vi "LFO Electrical Tests.vi"() -> ()   [LabVIEW 2018]
doc: "Use this template to build a producer/consumer design pattern with events to produce queue items. Use this design pattern instead of the User Interface Event Handler pattern for user interfaces when you want to execute code asynchronously in response to an event without slowing the user interface responsiveness."
uses:
  Custom Controls/LFO State Variable.ctl
  Custom Controls/BW NF State.ctl
  Custom Controls/Vitrek State Top.ctl
  Instrumentation/Door Status Global Variable.vi
  <vilib>/DAQmx/create/channels.llb/DAQmx Create Channel (DI-Digital Input).vi
panel:
  in  "base path":path=path "F:/Departments/Mfg Production/Shares/Plant2/LFO/125332 Electrical Test"
  out "Vitrek Stop?":bool
  out "BW2 Result Indicators":T1
  out "BW1 Result Indicators":T1
  out "BW 2 Results":T2
  out "BW 1 Results":T2
  out "Raw Data ACW BW1":T3
  out "Raw Data ACW BW2":T4
  in  "Vitrek State":T5
  out "No Fire Stop?":bool
  out "BW Stop?":bool
  out "Bridgewire 2 No-Fire":waveform(dbl)(graph)
  out "Bridgewire 1 No-Fire":waveform(dbl)(graph)
  out "No-Fire Results BW1":T6
  out "No-Fire Results BW2":T6
  in  "lower resistance limit":dbl=0.13
  in  "upper resistance limit":dbl=0.25
  out "BW 2 Resistance":string
  out "BW 1 Resistance":string
  out "Model # Out":string
  out "Serial # Out":string
  in  "BW State":T7
  out "Results Table":string[][](array[string])
  out "No-Fire Result":bool
  out "configuration file path":path=path "U:/Software Development/builds/LFO Electrical Tests/LFO Electrical Test/LFO Specifications.ini"
  in  "Tab Control":enum32{"Electrical Tests"}(tab)
  in  "Reset":bool
  out "Test Status":string
  out "Results":string[][](table)
  out "BW 1 Dielectric Strength Result":u16(ring)
  out "BW 2 Dielectric Strength Result":u16(ring)
  out "BW 1 Insulation Resistance Result":u16(ring)
  out "BW 2 Insulation Resistance Result":u16(ring)
  out "BW 1 Resistance Result":u16(ring)
  out "BW 2 Resistance Result":u16(ring)
  out "BW 1 No-Fire Result":u16(ring)
  out "BW 2 No-Fire Result":u16(ring)
  in  "stop":bool
  in  "Start Vitrek":bool=TRUE
  in  "Start BW":bool=TRUE
  out "Door Status":bool
  out "Raw Data Path":path
  in  "LFO State":T8=enum."Bridgewire"
  # "LFO Electrical Tests v2.0.2"
  # "Last Updated: 8/2/2022"
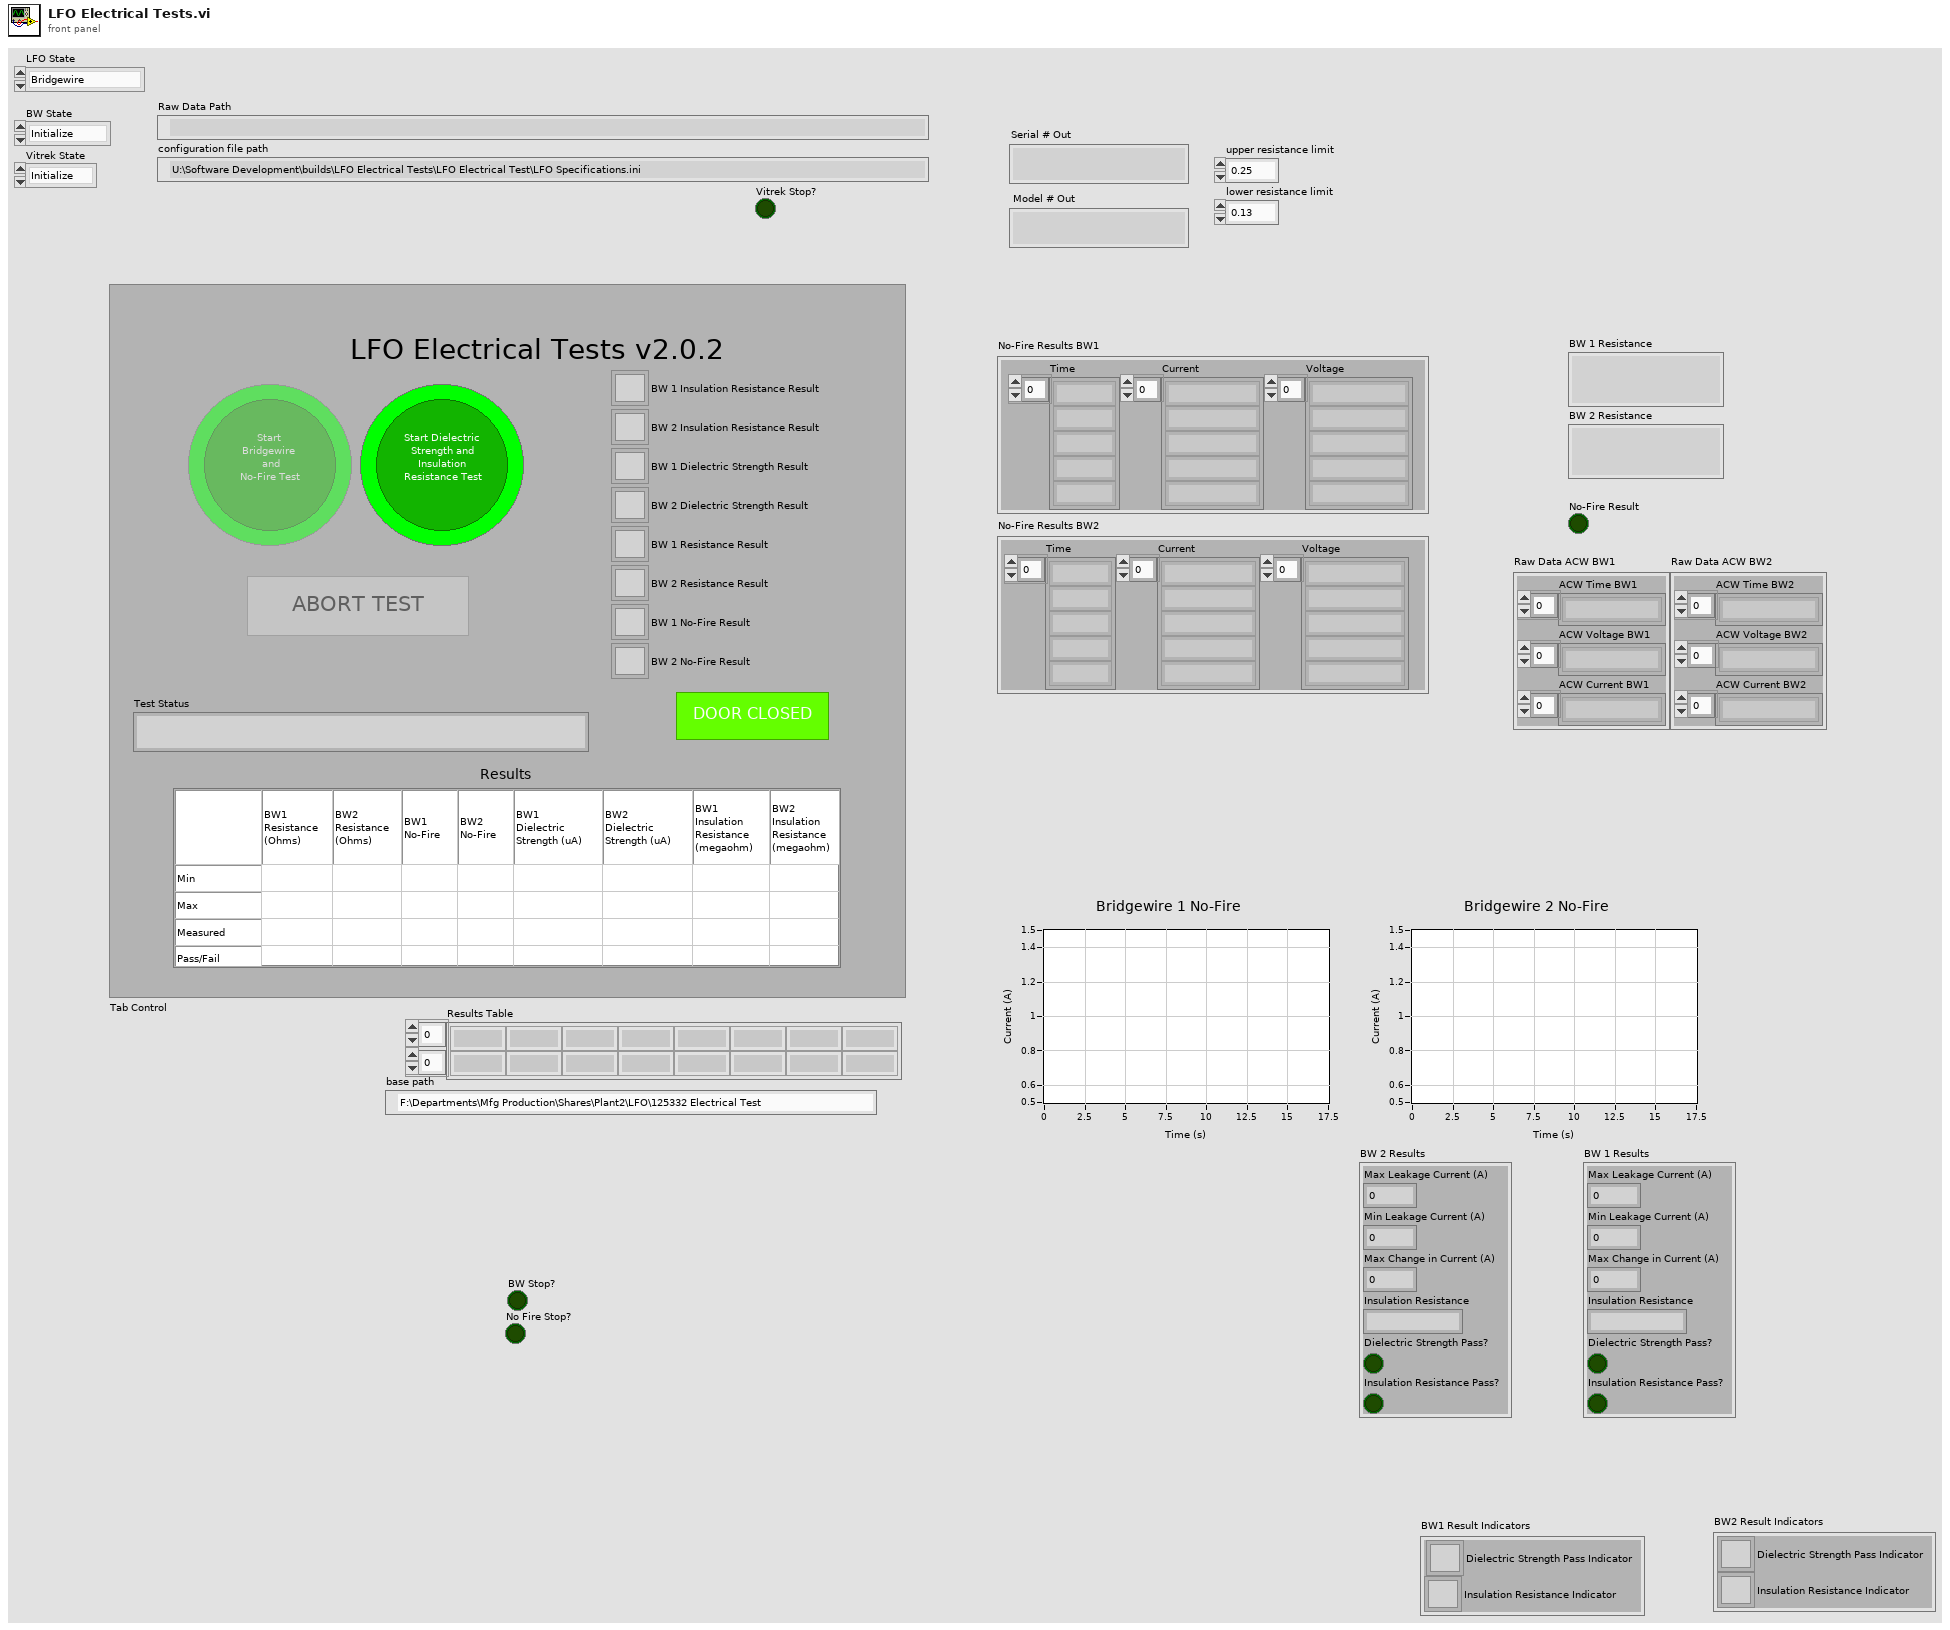
[diagram p1: front panel]
types:
  T1 = cluster{"Dielectric Strength Pass Indicator":u16, "Insulation Resistance Indicator":u16}
  T2 = cluster{"Max Leakage Current (A)":dbl, "Min Leakage Current (A)":dbl, "Max Change in Current (A)":dbl, "Dielectric Strength Pass?":bool, "Insulation Resistance Pass?":bool, "Insulation Resistance":string}
  T3 = cluster{"ACW Time BW1":string[], "ACW Voltage BW1":string[], "ACW Current BW1":string[]}
  T4 = cluster{"ACW Time BW2":string[], "ACW Voltage BW2":string[], "ACW Current BW2":string[]}
  T5 = typedef "Vitrek State Top.ctl" = enum16{"Initialize", "Run Vitrek", "End Vitrek"}
  T6 = cluster{"Current":string[], "Voltage":string[], "Time":string[]}
  T7 = typedef "BW NF State.ctl" = enum16{"Initialize", "Bridgewire Resistance", "No Fire Test", "End BW State"}
  T8 = typedef "LFO State Variable.ctl" = enum16{"Reset", "Bridgewire", "Switch Cable", "ACW and IR Test", "Report", "Exit"}
  T9 = cluster{"Instrument":string, "VISA resource name":refnum<visa-resource-name>}[]
  T10 = cluster{"BW1 Resistance (Ohms)":string, "BW2 Resistance (Ohms)":string, "BW1 No-Fire":string, "BW2 No-Fire":string, "BW1 Dielectric Strength (uA)":string, "BW2 Dielectric Strength (uA)":string, "BW1 Insulation Resistance (MOhms)":string, "BW2 Insulation Resistance (MOhms)":string}
  T11 = enum8{"Enabled", "Disabled", "Disabled and Grayed Out"}
  T12 = cluster{"BW 1 Resistance":string, "BW 2 Resistance":string, "No-Fire Results BW1":cluster{"Current":string[], "Voltage":string[], "Time":string[]}, "No-Fire Results BW2":cluster{"Current":string[], "Voltage":string[], "Time":string[]}, "ACW Results BW1":cluster{"ACW Time BW1":string[], "ACW Voltage BW1":string[], "ACW Current BW1":string[]}, "IR Results BW1":cluster{"Max Leakage Current (A)":dbl, "Min Leakage Current (A)":dbl, "Max Change in Current (A)":dbl, "Dielectric Strength Pass?":bool, "Insulation Resistance Pass?":bool, "Insulation Resistance":string}, "ACW Results BW2":cluster{"ACW Time BW2":string[], "ACW Voltage BW2":string[], "ACW Current BW2":string[]}, "IR Results BW 2":cluster{"Max Leakage Current (A)":dbl, "Min Leakage Current (A)":dbl, "Max Change in Current (A)":dbl, "Dielectric Strength Pass?":bool, "Insulation Resistance Pass?":bool, "Insulation Resistance":string}}
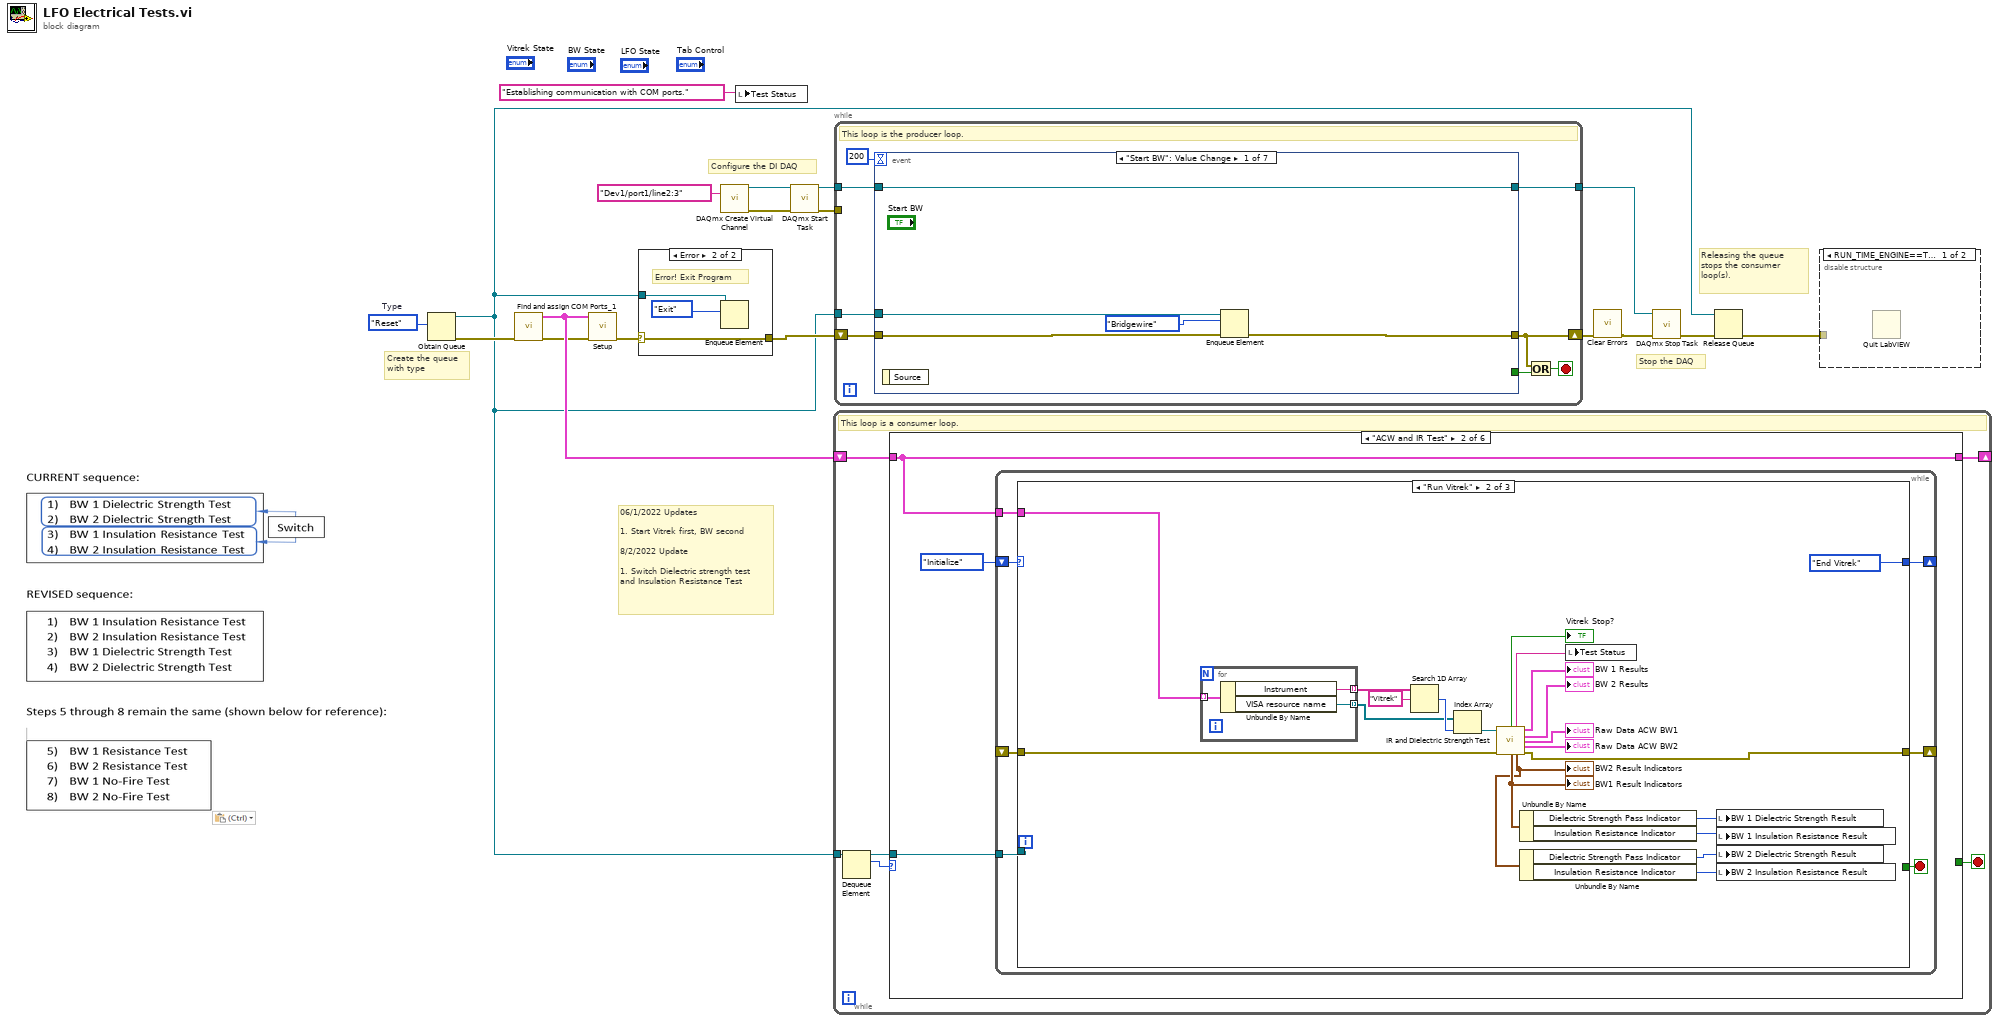
[diagram p0: block diagram]
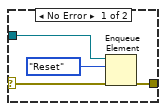
[diagram p3: hidden frame]
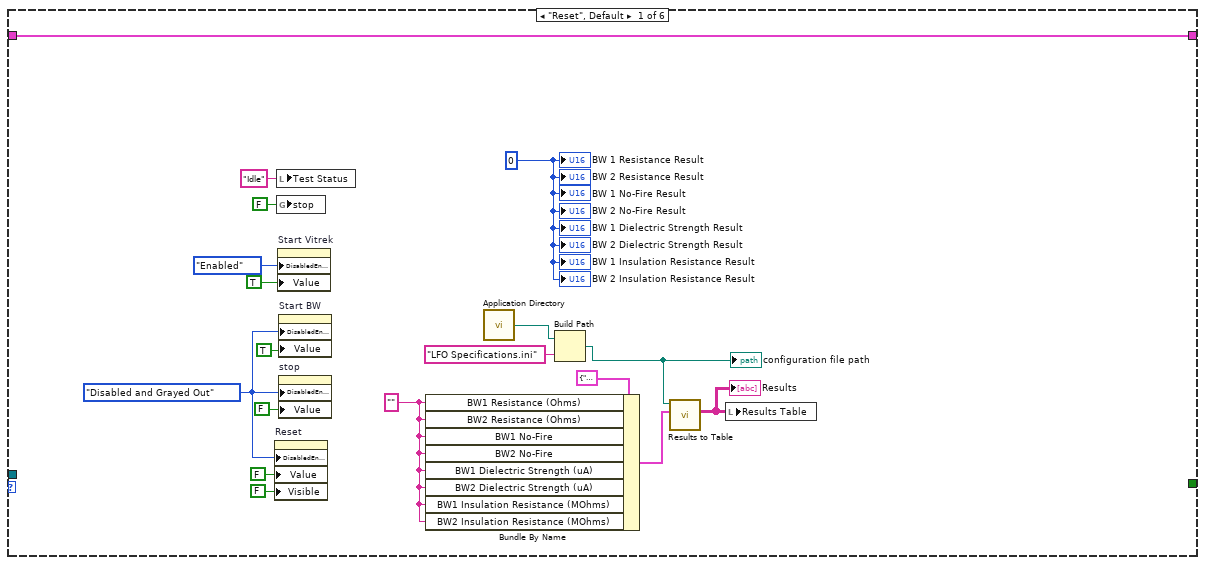
[diagram p4: hidden frame]
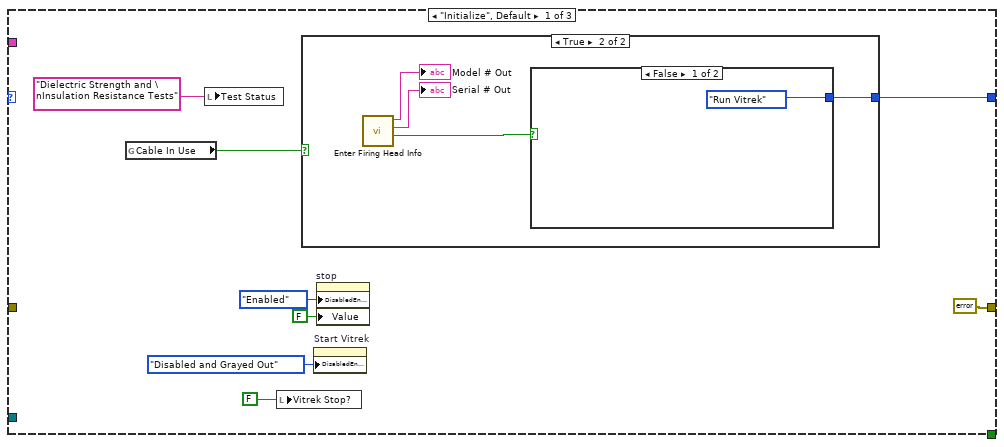
[diagram p5: hidden frame]
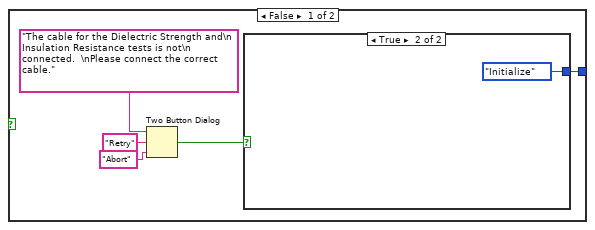
[diagram p6: hidden frame]
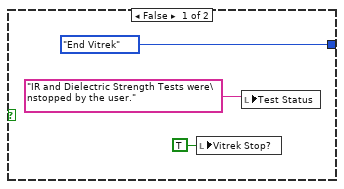
[diagram p7: hidden frame]
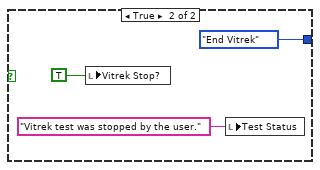
[diagram p8: hidden frame]
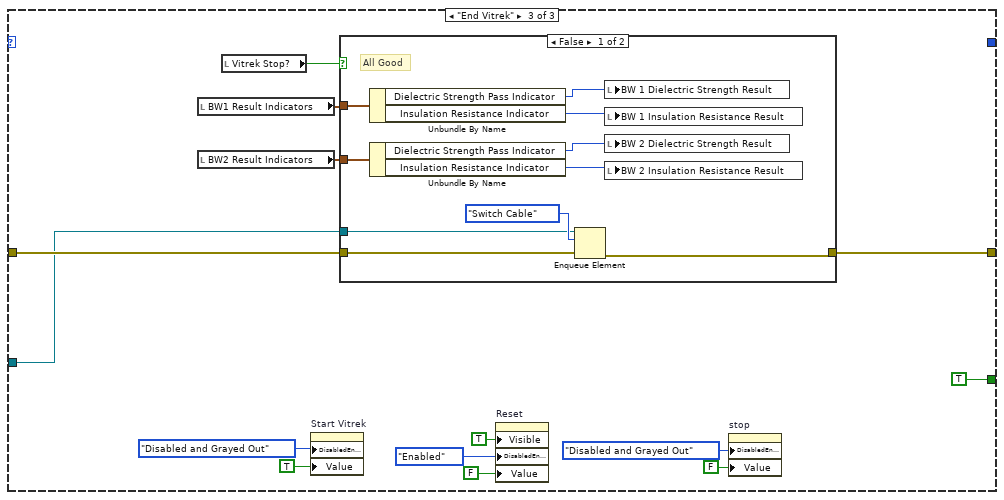
[diagram p9: hidden frame]
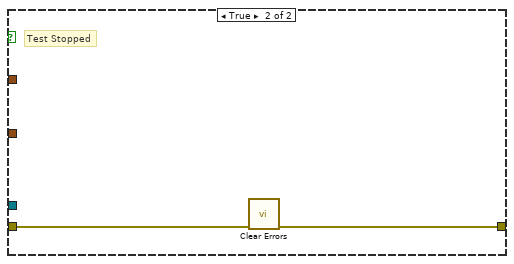
[diagram p10: hidden frame]
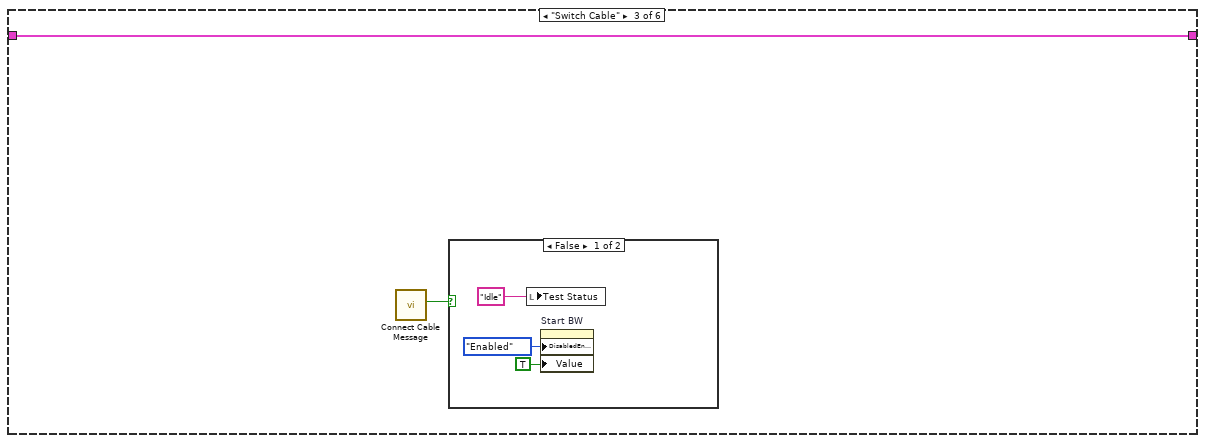
[diagram p11: hidden frame]
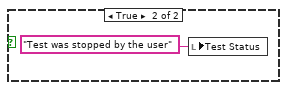
[diagram p12: hidden frame]
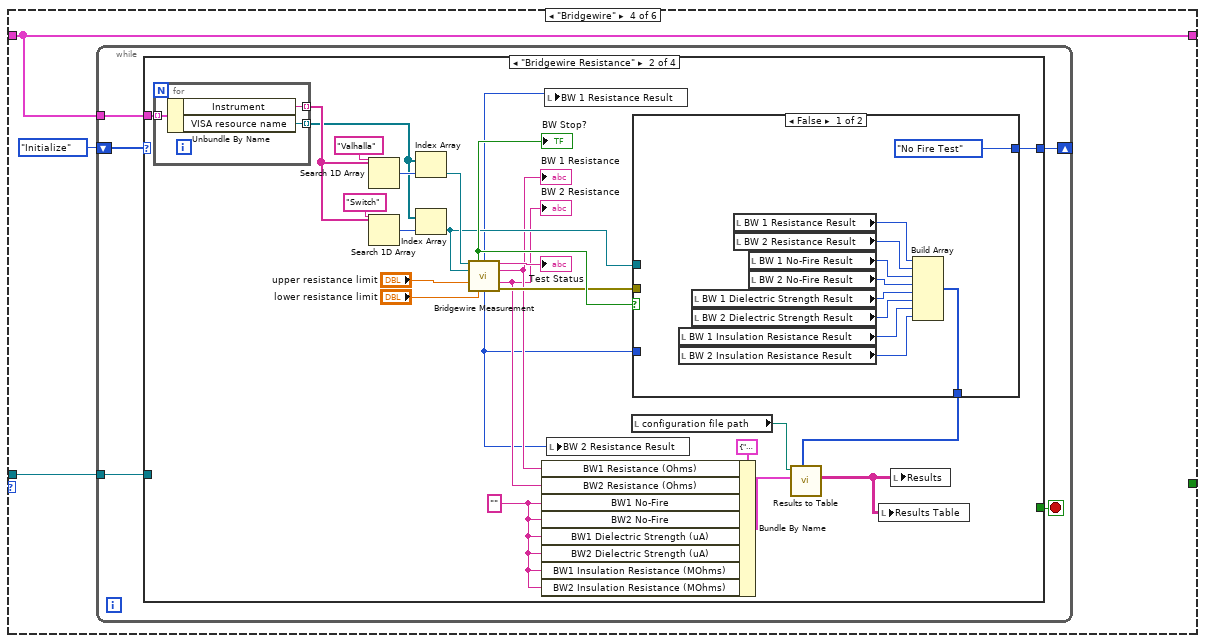
[diagram p13: hidden frame]
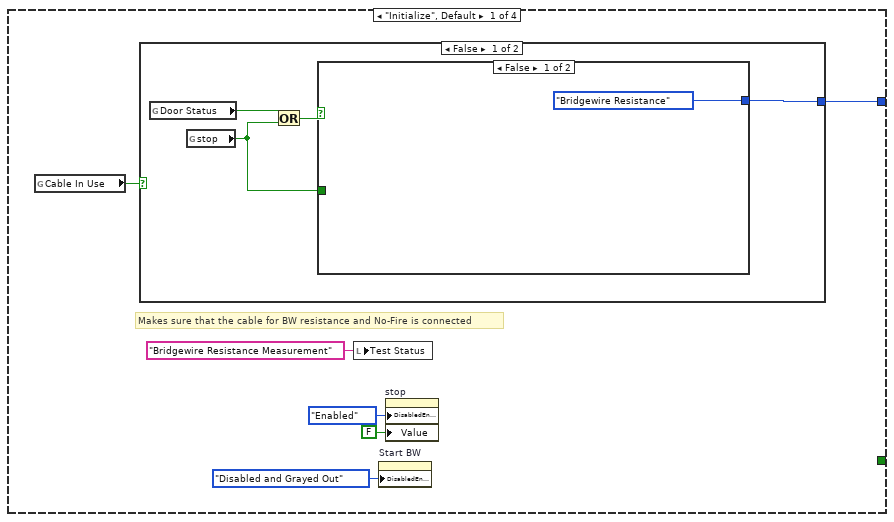
[diagram p14: hidden frame]
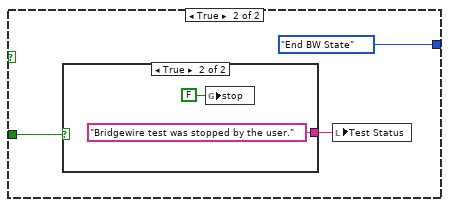
[diagram p15: hidden frame]
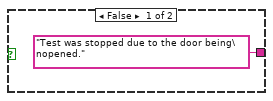
[diagram p16: hidden frame]
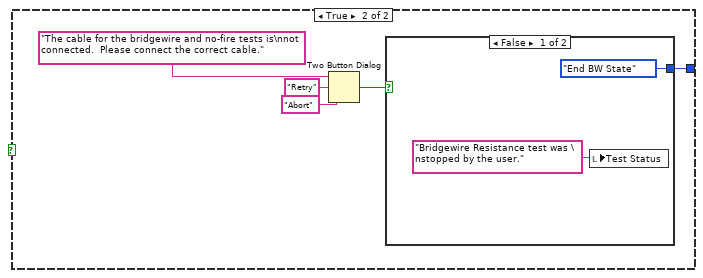
[diagram p17: hidden frame]
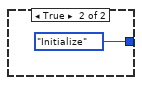
[diagram p18: hidden frame]
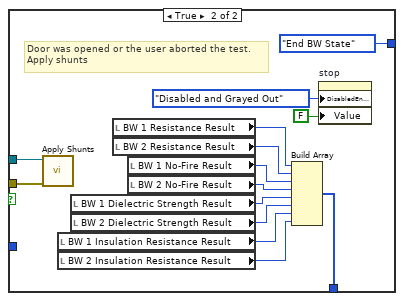
[diagram p19: hidden frame]
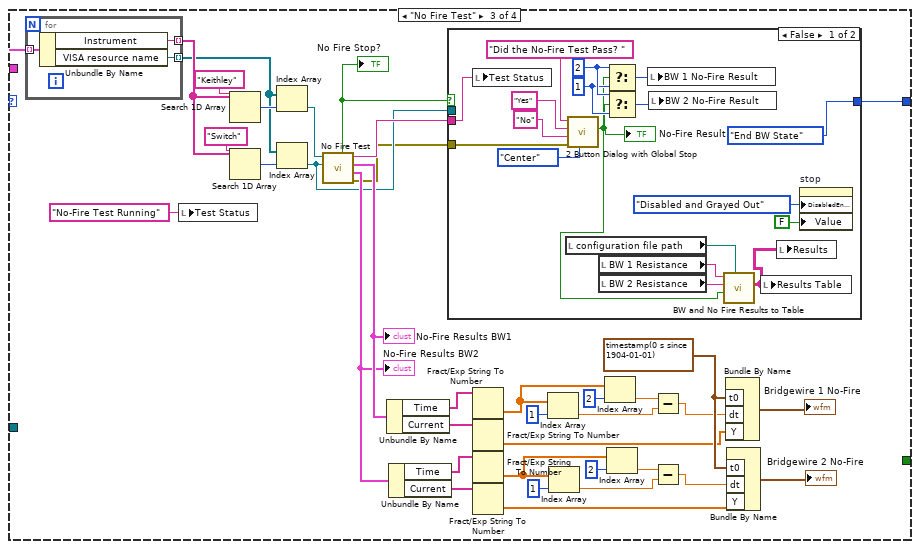
[diagram p20: hidden frame]
diagram:
  w18 = LFO_State_Variable."Reset"  # Type
  # "Stop the DAQ"
  # "Configure the DI DAQ"
  # "Create the queue\nwith type"
  # "06/1/2022 Updates\n\n1. Start Vitrek first, BW second\n\n8/2/2022 Update\n\n1. Switch Dielectric strength test\nand Insulation Resistance Test"
  # "Releasing the queue stops the consumer loop(s)."
  n1 = Obtain Queue(element data type=w18) -> (queue out=w10:refnum<queue>, error out=w11:errorcluster)  [unwired: 4 in, 1 out]
  n2 = call "Find and assign COM Ports_1.vi"("error in (no error)"=w11) -> ("error out"=w1:errorcluster, "Assigned VISA Ports"=w16:T9)  [unwired: 8 in, 1 out]
  n3 = call "Setup.vi"("error in (no error)"=w1, "Assigned VISA Ports"=w16) -> ("error out"=w6:errorcluster)  [unwired: 9 in]
  n4 = case shown="Error" w6 {
    selector: w6 -> [w21 w22]
    tunnel: [w21 w22] -> w17
    tunnel: w10 -> [w19 w24]
    frame No Error {
      n5 = Enqueue Element(queue=w19, element=LFO_State_Variable."Reset") -> ()  [unwired: 2 in, 3 out]
    }
    frame Error {
      # "Error! Exit Program"
      n6 = Enqueue Element(queue=w24, element=LFO_State_Variable."Exit") -> ()  [unwired: 2 in, 3 out]
    }
  }
  n7 = call-poly <vilib>:"DAQmx Create Virtual Channel.vi"("lines"=tag "Dev1/port1/line2:3" ("Door Status Input")) -> ("task out"=w8:refnum<k21>, "error out"=w9:errorcluster)  [unwired: 13 in]
  n8 = local write "Test Status"("Establishing communication with COM ports." ("Test Status")) -> ()
  n9 = call <vilib>:"DAQmx Start Task.vi"("task/channels in"=w8, "error in"=w9) -> ("task out"=w15:refnum<k21>, "error out"=w2:errorcluster)  [unwired: 12 in]
  n10 = while {
    tunnel: w10 -> [w30]
    shift-right: [w26] -> _
    shift-left: w16 -> [w27]
    stop <- w28 stop-if-true
    # "This loop is a consumer loop."
    n11 = Dequeue Element(queue=w30) -> (queue out=w25:refnum<queue>, element=w29:T8)  [unwired: 2 in, 2 out]
    n12 = case shown="\"ACW and IR Test\"" w29 {
      tunnel: w27 -> [w48 w50 w135 w142 w353 w354]
      tunnel: [_ _ _ _ _ TRUE] -> w28
      tunnel: [w48 w50 w135 w142 w353 w354] -> w26
      tunnel: w25 -> [_ w49 _ w140 _ _]
      frame "Reset", Default {
        w32 = u16 0 ("BW 1 Resistance Result")
        w31 = T11."Disabled and Grayed Out" ("Disabled")
        w41 = "" ("BW1 Resistance (Ohms)")
        n13 = property on="Reset" class="Bool (strict)"("DisabledEnum"=w31, "Value"=FALSE ("stop"), "Visible"=FALSE) -> ()  [unwired: 2 in, 2 out]
        n14 = local write "Test Status"("Idle" ("Test Status")) -> ()
        n15 = global write "Door Status Global Variable.vi" "stop"(FALSE ("stop")) -> ()
        n16 = property on="Start Vitrek" class="Bool (strict)"("DisabledEnum"=T11."Enabled" ("Disabled"), "Value"=TRUE ("stop")) -> ()  [unwired: 2 in, 2 out]
        n17 = property on="Start BW" class="Bool (strict)"("DisabledEnum"=w31, "Value"=TRUE ("stop")) -> ()  [unwired: 2 in, 2 out]
        n18 = property on="stop" class="Bool (strict)"("DisabledEnum"=w31, "Value"=FALSE ("stop")) -> ()  [unwired: 2 in, 2 out]
        n19 = Bundle By Name(cluster=T10 {"BW1 Resistance (Ohms)"="4870 ", "BW2 Resistance (Ohms)"="4870 ", "BW1 No-Fire"="4870 ", "BW2 No-Fire"="4870 ", "BW1 Dielectric Strength (uA)"="4870 ", "BW2 Dielectric Strength (uA)"="4870 ", "BW1 Insulation Resistance (MOhms)"="4870 ", "BW2 Insulation Resistance (MOhms)"="4870 "} ("Test Results"), "BW1 Resistance (Ohms)"=w41, "BW2 Resistance (Ohms)"=w41, "BW1 No-Fire"=w41, "BW2 No-Fire"=w41, "BW1 Dielectric Strength (uA)"=w41, "BW2 Dielectric Strength (uA)"=w41, "BW1 Insulation Resistance (MOhms)"=w41, "BW2 Insulation Resistance (MOhms)"=w41) -> (w43:T10)
        n20 = call <vilib>:"Application Directory.vi"() -> ("Application Directory"=w38:path)
        n21 = Build Path(base path=w38, name or relative path="LFO Specifications.ini") -> (appended path=w36:path)
        "configuration file path" <- w36
        n22 = call "Results to Table.vi"("Test Results"=w43, "configuration file path"=w36) -> ("Results Table"=w39:string[][])  [unwired: 8 in, 1 out]
        "Results" <- w39
        n23 = local write "Results Table"(w39) -> ()
        "BW 1 Dielectric Strength Result" <- w32
        "BW 2 Dielectric Strength Result" <- w32
        "BW 1 Insulation Resistance Result" <- w32
        "BW 2 Insulation Resistance Result" <- w32
        "BW 1 Resistance Result" <- w32
        "BW 2 Resistance Result" <- w32
        "BW 1 No-Fire Result" <- w32
        "BW 2 No-Fire Result" <- w32
      }
      frame "ACW and IR Test" {
        n24 = while {
          shift-right: [w57] -> _
          shift-left: Vitrek_State_Top."Initialize" ("Vitrek State") -> [w58]
          tunnel: w50 -> [w56]
          shift-right: [w55] -> _
          shift-left: _ -> [w54]
          tunnel: w49 -> [w52]
          stop <- w53 stop-if-true
          n25 = case shown="\"Run Vitrek\"" w58 {
            tunnel: [w66 Vitrek_State_Top."End Vitrek" ("Vitrek State") _] -> w57
            tunnel: w56 -> [_ w100 _]
            tunnel: [errorcluster {"status"=FALSE, "code"=0, "source"=""} ("error in (no error)") w92 w108] -> w55
            tunnel: w54 -> [_ w98 w121]
            tunnel: [_ _ TRUE] -> w53
            tunnel: w52 -> [_ _ w109]
            frame "Initialize", Default {
              n26 = global read "Door Status Global Variable.vi" "Cable In Use"() -> (w60:bool)
              n27 = local write "Test Status"("Dielectric Strength and \nInsulation Resistance Tests" ("Test Status")) -> ()
              n28 = local write "Vitrek Stop?"(FALSE ("Vitrek Init Stop?")) -> ()
              n29 = case shown="True" w60 {
                tunnel: [w68 w79] -> w66
                frame False {
                  n30 = Two Button Dialog(message="The cable for the Dielectric Strength and\n Insulation Resistance tests is not\n connected.  \nPlease connect the correct cable.", 1:"Abort" ("F button name (\"Cancel\")"), 2:"Retry" ("T button name (\"OK\")")) -> (T button?=w67:bool)
                  n31 = case shown="True" w67 {
                    tunnel: [Vitrek_State_Top."End Vitrek" ("Vitrek State") Vitrek_State_Top."Initialize" ("Vitrek State")] -> w68
                    frame False {
                      n32 = local write "Vitrek Stop?"(TRUE ("Vitrek Stop?")) -> ()
                      n33 = local write "Test Status"("IR and Dielectric Strength Tests were\nstopped by the user." ("Test Status")) -> ()
                    }
                    frame True {
                    }
                  }
                }
                frame True {
                  n34 = call "Enter Firing Head Info.vi"() -> ("Abort Test?"=w76:bool, "Serial # Out"=→"Serial # Out":string, "Model # Out"=→"Model # Out":string)  [unwired: 7 in, 1 out]
                  n35 = case shown="False" w76 {
                    tunnel: [Vitrek_State_Top."Run Vitrek" ("Vitrek State") Vitrek_State_Top."End Vitrek" ("Vitrek State")] -> w79
                    frame False {
                    }
                    frame True {
                      n36 = local write "Vitrek Stop?"(TRUE ("Vitrek Init Stop?")) -> ()
                      n37 = local write "Test Status"("Vitrek test was stopped by the user." ("Test Status")) -> ()
                    }
                  }
                }
              }
              n38 = property on="Start Vitrek" class="Bool (strict)"("DisabledEnum"=T11."Disabled and Grayed Out" ("Disabled")) -> ()  [unwired: 2 in, 2 out]
              n39 = property on="stop" class="Bool (strict)"("DisabledEnum"=T11."Enabled" ("Disabled"), "Value"=FALSE ("stop")) -> ()  [unwired: 2 in, 2 out]
            }
            frame "Run Vitrek" {
              n40 = for {
                tunnel: w100 -> [w107] mode=indexing
                tunnel: [w106] -> w102 mode=indexing
                tunnel: [w105] -> w101 mode=indexing
                n41 = Unbundle By Name(w107) -> ("Instrument"=w106:string, "VISA resource name"=w105:refnum<visa-resource-name>)
              }
              n42 = Search 1D Array(1D array=w102, element="Vitrek") -> (index of element=w103:i32)  [unwired: 1 in]
              n43 = Index Array(array=w101, index=w103) -> (element=w90:refnum<visa-resource-name>)
              n44 = call "IR and Dielectric Strength Test.vi"("VISA resource name in"=w90, "error in (no error)"=w98) -> (2:"Stop Status"=→"Vitrek Stop?":bool, 3:"Stop Status"=w96:string, "BW 1 Results"=→"BW 1 Results":T2, "BW 2 Results"=→"BW 2 Results":T2, "Raw Data ACW BW1"=→"Raw Data ACW BW1":T3, "Raw Data ACW BW2"=→"Raw Data ACW BW2":T4, "BW1 Result Indicators"=w85:T1, "BW2 Result Indicators"=w84:T1, "error out"=w92:errorcluster)  [unwired: 5 in]
              "BW2 Result Indicators" <- w84
              "BW1 Result Indicators" <- w85
              n45 = Unbundle By Name(w85) -> ("Dielectric Strength Pass Indicator"=w87:u16, "Insulation Resistance Indicator"=w86:u16)
              n46 = Unbundle By Name(w84) -> ("Dielectric Strength Pass Indicator"=w89:u16, "Insulation Resistance Indicator"=w88:u16)
              n47 = local write "Test Status"(w96) -> ()
              n48 = local write "BW 1 Dielectric Strength Result"(w87) -> ()
              n49 = local write "BW 1 Insulation Resistance Result"(w86) -> ()
              n50 = local write "BW 2 Dielectric Strength Result"(w89) -> ()
              n51 = local write "BW 2 Insulation Resistance Result"(w88) -> ()
            }
            frame "End Vitrek" {
              n52 = local read "BW1 Result Indicators"() -> (w111:T1)
              n53 = local read "BW2 Result Indicators"() -> (w110:T1)
              n54 = local read "Vitrek Stop?"() -> (w112:bool)
              n55 = property on="Start Vitrek" class="Bool (strict)"("DisabledEnum"=T11."Disabled and Grayed Out" ("Disabled"), "Value"=TRUE ("stop")) -> ()  [unwired: 2 in, 2 out]
              n56 = case shown="False" w112 {
                tunnel: w110 -> [w131 _]
                tunnel: w111 -> [w130 _]
                tunnel: [w122 w132] -> w108
                tunnel: w121 -> [w123 w133]
                tunnel: w109 -> [w124 _]
                frame False {
                  # "All Good"
                  n57 = Unbundle By Name(w130) -> ("Dielectric Strength Pass Indicator"=w129:u16, "Insulation Resistance Indicator"=w128:u16)
                  n58 = Unbundle By Name(w131) -> ("Dielectric Strength Pass Indicator"=w127:u16, "Insulation Resistance Indicator"=w126:u16)
                  n59 = Enqueue Element(queue=w124, element=LFO_State_Variable."Switch Cable", error in (no error)=w123) -> (error out=w122:errorcluster)  [unwired: 1 in, 2 out]
                  n60 = local write "BW 1 Dielectric Strength Result"(w129) -> ()
                  n61 = local write "BW 1 Insulation Resistance Result"(w128) -> ()
                  n62 = local write "BW 2 Dielectric Strength Result"(w127) -> ()
                  n63 = local write "BW 2 Insulation Resistance Result"(w126) -> ()
                }
                frame True {
                  # "Test Stopped"
                  n64 = call <vilib>:"Clear Errors.vi"("error in (no error)"=w133) -> ("error out"=w132:errorcluster)  [unwired: 5 in, 1 out]
                }
              }
              n65 = property on="Reset" class="Bool (strict)"("Visible"=TRUE, "DisabledEnum"=T11."Enabled" ("Disabled"), "Value"=FALSE ("Start BW")) -> ()  [unwired: 2 in, 2 out]
              n66 = property on="stop" class="Bool (strict)"("DisabledEnum"=T11."Disabled and Grayed Out" ("Disabled"), "Value"=FALSE ("Start BW")) -> ()  [unwired: 2 in, 2 out]
            }
          }
        }
      }
      frame "Switch Cable" {
        n67 = call "Connect Cable Message.vi"() -> ("Aborted?"=w134:bool)  [unwired: 10 in, 1 out]
        n68 = case shown="False" w134 {
          frame False {
            n69 = local write "Test Status"("Idle" ("Test Status")) -> ()
            n70 = property on="Start BW" class="Bool (strict)"("DisabledEnum"=T11."Enabled" ("Disabled"), "Value"=TRUE ("Start BW")) -> ()  [unwired: 2 in, 2 out]
          }
          frame True {
            n71 = local write "Test Status"("Test was stopped by the user" ("Test Status")) -> ()
          }
        }
      }
      frame "Bridgewire" {
        n72 = while {
          shift-right: [w146] -> _
          shift-left: BW_NF_State."Initialize" ("BW State") -> [w147]
          tunnel: w142 -> [w145]
          tunnel: w140 -> [w143]
          stop <- w144 stop-if-true
          n73 = case shown="\"Bridgewire Resistance\"" w147 {
            tunnel: [w153 w184 w235 _] -> w146
            tunnel: w145 -> [_ w189 w241 _]
            tunnel: [_ _ _ TRUE] -> w144
            tunnel: w143 -> [_ _ _ w294]
            frame "Initialize", Default {
              # "Makes sure that the cable for BW resistance and No-Fire is connected"
              n74 = global read "Door Status Global Variable.vi" "Cable In Use"() -> (w152:bool)
              n75 = case shown="False" w152 {
                tunnel: [w154 w166] -> w153
                frame False {
                  n76 = global read "Door Status Global Variable.vi" "Door Status"() -> (w157:bool)
                  n77 = global read "Door Status Global Variable.vi" "stop"() -> (w156:bool)
                  n78 = Or(x=w157, y=w156) -> (x .or. y?=w155:bool)
                  n79 = case shown="False" w155 {
                    tunnel: w156 -> [_ w161]
                    tunnel: [BW_NF_State."Bridgewire Resistance" ("BW State") BW_NF_State."End BW State" ("BW State")] -> w154
                    frame False {
                    }
                    frame True {
                      n80 = case shown="True" w161 {
                        tunnel: ["Test was stopped due to the door being\nopened." ("Test Status") "Bridgewire test was stopped by the user." ("Test Status")] -> w160
                        frame False {
                        }
                        frame True {
                          n81 = global write "Door Status Global Variable.vi" "stop"(FALSE ("stop")) -> ()
                        }
                      }
                      n82 = local write "Test Status"(w160) -> ()
                    }
                  }
                }
                frame True {
                  n83 = Two Button Dialog(message="The cable for the bridgewire and no-fire tests is\nnot connected.  Please connect the correct cable.", 1:"Abort" ("F button name (\"Cancel\")"), 2:"Retry" ("T button name (\"OK\")")) -> (T button?=w165:bool)
                  n84 = case shown="False" w165 {
                    tunnel: [BW_NF_State."End BW State" ("BW State") BW_NF_State."Initialize" ("BW State")] -> w166
                    frame False {
                      n85 = local write "Test Status"("Bridgewire Resistance test was \nstopped by the user." ("Test Status")) -> ()
                    }
                    frame True {
                    }
                  }
                }
              }
              n86 = local write "Test Status"("Bridgewire Resistance Measurement" ("Test Status")) -> ()
              n87 = property on="Start BW" class="Bool (strict)"("DisabledEnum"=T11."Disabled and Grayed Out" ("Disabled")) -> ()  [unwired: 2 in, 2 out]
              n88 = property on="stop" class="Bool (strict)"("DisabledEnum"=T11."Enabled" ("Disabled"), "Value"=FALSE ("stop")) -> ()  [unwired: 2 in, 2 out]
            }
            frame "Bridgewire Resistance" {
              w176 = "" ("BW1 No-Fire")
              n89 = for {
                tunnel: w189 -> [w224] mode=indexing
                tunnel: [w223] -> w190 mode=indexing
                tunnel: [w222] -> w188 mode=indexing
                n90 = Unbundle By Name(w224) -> ("Instrument"=w223:string, "VISA resource name"=w222:refnum<visa-resource-name>)
              }
              n91 = Search 1D Array(1D array=w190, element="Valhalla") -> (index of element=w193:i32)  [unwired: 1 in]
              n92 = Search 1D Array(1D array=w190, element="Switch") -> (index of element=w191:i32)  [unwired: 1 in]
              n93 = Index Array(array=w188, index=w193) -> (element=w187:refnum<visa-resource-name>)
              n94 = Index Array(array=w188, index=w191) -> (element=w183:refnum<visa-resource-name>)
              n95 = call "Bridgewire Measurement.vi"("Valhalla Resource Name"=w187, "Switch Resource Name"=w183, "upper resistance limit"="upper resistance limit", "lower resistance limit"="lower resistance limit") -> ("Stop Status"=w186:bool, "BW1 Resistance Result"=w173:u16, "Test Status"=→"Test Status":string, "BW 1 Resistance"=w179:string, "BW 2 Resistance"=w178:string, "BW2 Resistance Result"=w174:u16, "error out"=w185:errorcluster)  [unwired: 3 in, 2 out]
              "BW 1 Resistance" <- w179
              "BW 2 Resistance" <- w178
              "BW Stop?" <- w186
              n96 = Bundle By Name(cluster=T10 {"BW1 Resistance (Ohms)"="4870 ", "BW2 Resistance (Ohms)"="4870 ", "BW1 No-Fire"="4870 ", "BW2 No-Fire"="4870 ", "BW1 Dielectric Strength (uA)"="4870 ", "BW2 Dielectric Strength (uA)"="4870 ", "BW1 Insulation Resistance (MOhms)"="4870 ", "BW2 Insulation Resistance (MOhms)"="4870 "} ("Test Results"), "BW1 Resistance (Ohms)"=w179, "BW2 Resistance (Ohms)"=w178, "BW1 No-Fire"=w176, "BW2 No-Fire"=w176, "BW1 Dielectric Strength (uA)"=w176, "BW2 Dielectric Strength (uA)"=w176, "BW1 Insulation Resistance (MOhms)"=w176, "BW2 Insulation Resistance (MOhms)"=w176) -> (w181:T10)
              n97 = local write "BW 1 Resistance Result"(w173) -> ()
              n98 = local write "BW 2 Resistance Result"(w174) -> ()
              n99 = local read "configuration file path"() -> (w180:path)
              n100 = case shown="False" w186 {
                tunnel: w185 -> [_ w219]
                tunnel: [BW_NF_State."No Fire Test" ("BW State") BW_NF_State."End BW State" ("BW State")] -> w184
                tunnel: w183 -> [_ w217]
                tunnel: [w198 w208] -> w175
                tunnel: w174 -> [_ _]
                frame False {
                  n101 = local read "BW 1 Insulation Resistance Result"() -> (w200:u16)
                  n102 = local read "BW 2 Insulation Resistance Result"() -> (w199:u16)
                  n103 = local read "BW 1 Dielectric Strength Result"() -> (w202:u16)
                  n104 = local read "BW 2 Dielectric Strength Result"() -> (w201:u16)
                  n105 = local read "BW 1 Resistance Result"() -> (w206:u16)
                  n106 = local read "BW 2 Resistance Result"() -> (w205:u16)
                  n107 = local read "BW 1 No-Fire Result"() -> (w204:u16)
                  n108 = local read "BW 2 No-Fire Result"() -> (w203:u16)
                  n109 = Build Array(w206, w205, w204, w203, w202, w201, w200, w199) -> (w198:u16[])
                }
                frame True {
                  # "Door was opened or the user aborted the test.\nApply shunts"
                  n110 = call "Apply Shunts.vi"("error in (no error)"=w219, "VISA Refnum in"=w217) -> ()  [unwired: 9 in, 1 out]
                  n111 = local read "BW 1 Insulation Resistance Result"() -> (w210:u16)
                  n112 = local read "BW 2 Insulation Resistance Result"() -> (w209:u16)
                  n113 = local read "BW 1 Dielectric Strength Result"() -> (w212:u16)
                  n114 = local read "BW 2 Dielectric Strength Result"() -> (w211:u16)
                  n115 = local read "BW 1 Resistance Result"() -> (w216:u16)
                  n116 = local read "BW 2 Resistance Result"() -> (w215:u16)
                  n117 = local read "BW 1 No-Fire Result"() -> (w214:u16)
                  n118 = local read "BW 2 No-Fire Result"() -> (w213:u16)
                  n119 = Build Array(w216, w215, w214, w213, w212, w211, w210, w209) -> (w208:u16[])
                  n120 = property on="stop" class="Bool (strict)"("DisabledEnum"=T11."Disabled and Grayed Out" ("Disabled"), "Value"=FALSE ("Start BW")) -> ()  [unwired: 2 in, 2 out]
                }
              }
              n121 = call "Results to Table.vi"("Result Indicators"=w175, "Test Results"=w181, "configuration file path"=w180) -> ("Results Table"=w177:string[][])  [unwired: 7 in, 1 out]
              n122 = local write "Results Table"(w177) -> ()
              n123 = local write "Results"(w177) -> ()
            }
            frame "No Fire Test" {
              w254 = timestamp(0 s since 1904-01-01) ("t0")
              n124 = for {
                tunnel: w241 -> [w288] mode=indexing
                tunnel: [w287] -> w243 mode=indexing
                tunnel: [w286] -> w242 mode=indexing
                n125 = Unbundle By Name(w288) -> ("Instrument"=w287:string, "VISA resource name"=w286:refnum<visa-resource-name>)
              }
              n126 = local write "Test Status"("No-Fire Test Running" ("Test Status")) -> ()
              n127 = Search 1D Array(1D array=w243, element="Keithley") -> (index of element=w246:i32)  [unwired: 1 in]
              n128 = Search 1D Array(1D array=w243, element="Switch") -> (index of element=w244:i32)  [unwired: 1 in]
              n129 = Index Array(array=w242, index=w246) -> (element=w240:refnum<visa-resource-name>)
              n130 = Index Array(array=w242, index=w244) -> (element=w237:refnum<visa-resource-name>)
              n131 = call "No Fire Test.vi"("Switch Resource Name"=w237, "Keithley Resource Name"=w240) -> ("error out"=w236:errorcluster, "No-Fire Results BW2"=w248:T6, "No-Fire Results BW1"=w249:T6, "Test Status"=w238:string, "Stop Status"=w239:bool)  [unwired: 5 in]
              "No-Fire Results BW2" <- w248
              "No-Fire Results BW1" <- w249
              "No Fire Stop?" <- w239
              n132 = Unbundle By Name(w249) -> ("Time"=w260:string[], "Current"=w259:string[])
              n133 = Unbundle By Name(w248) -> ("Time"=w258:string[], "Current"=w257:string[])
              n134 = case shown="False" w239 {
                tunnel: w236 -> [w275 w284]
                tunnel: w238 -> [w270 w285]
                tunnel: w237 -> [_ w283]
                tunnel: [BW_NF_State."End BW State" ("BW State") BW_NF_State."End BW State" ("BW State")] -> w235
                frame False {
                  w277 = u16 1 ("BW 1 Resistance Result")
                  w279 = u16 2 ("BW 1 Resistance Result")
                  n135 = local write "Test Status"(w270) -> ()
                  n136 = local read "configuration file path"() -> (w264:path)
                  n137 = call "2 Button Dialog with Global Stop.vi"("Text.Justification"=enum16{"Left", "Center", "Right"}."Center", "error in (no error)"=w275, "F Button Name (\"CANCEL\")"="No" ("F button name (\"Cancel\")"), "T Button Name (\"OK\")"="Yes" ("T button name (\"OK\")"), "Dialog Message"="Did the No-Fire Test Pass? " ("message")) -> ("result"=w262:bool)  [unwired: 4 in, 2 out]
                  "No-Fire Result" <- w262
                  n138 = local read "BW 1 Resistance"() -> (w265:string)
                  n139 = local read "BW 2 Resistance"() -> (w266:string)
                  n140 = Select(t=w279, s=w262, f=w277) -> (s? t:f=w278:u16)
                  n141 = Select(t=w279, s=w262, f=w277) -> (s? t:f=w276:u16)
                  n142 = local write "BW 1 No-Fire Result"(w278) -> ()
                  n143 = local write "BW 2 No-Fire Result"(w276) -> ()
                  n144 = call "BW and No Fire Results to Table.vi"("configuration file path"=w264, "No-Fire Result"=w262, "BW 2 Resistance"=w266, "BW 1 Resistance"=w265) -> ("Results Table"=w263:string[][])  [unwired: 6 in, 1 out]
                  n145 = local write "Results Table"(w263) -> ()
                  n146 = local write "Results"(w263) -> ()
                  n147 = property on="stop" class="Bool (strict)"("DisabledEnum"=T11."Disabled and Grayed Out" ("Disabled"), "Value"=FALSE ("Start BW")) -> ()  [unwired: 2 in, 2 out]
                }
                frame True {
                  # "Door was opened or the user \naborted the test.\nApply shunts and initialize \ncontrols"
                  n148 = local write "Test Status"(w285) -> ()
                  n149 = call "Apply Shunts.vi"("error in (no error)"=w284, "VISA Refnum in"=w283) -> ()  [unwired: 9 in, 1 out]
                  n150 = property on="stop" class="Bool (strict)"("DisabledEnum"=T11."Disabled and Grayed Out" ("Disabled"), "Value"=FALSE ("Start BW")) -> ()  [unwired: 2 in, 2 out]
                }
              }
              n151 = Fract/Exp String To Number(string=w260) -> (number=w231:dbl[])  [unwired: 3 in, 1 out]
              n152 = Fract/Exp String To Number(string=w259) -> (number=w252:dbl[])  [unwired: 3 in, 1 out]
              n153 = Fract/Exp String To Number(string=w258) -> (number=w232:dbl[])  [unwired: 3 in, 1 out]
              n154 = Fract/Exp String To Number(string=w257) -> (number=w255:dbl[])  [unwired: 3 in, 1 out]
              n155 = Index Array(array=w231, index=1) -> (element=w228:dbl)
              n156 = Index Array(array=w232, index=1) -> (element=w227:dbl)
              n157 = Index Array(array=w231, index=2) -> (element=w230:dbl)
              n158 = Index Array(array=w232, index=2) -> (element=w229:dbl)
              n159 = Subtract(x=w230, y=w228) -> (x-y=w226:dbl)
              n160 = Subtract(x=w229, y=w227) -> (x-y=w225:dbl)
              n161 = Bundle By Name("t0"=w254, "dt"=w226, "Y"=w252) -> (→"Bridgewire 1 No-Fire":waveform(dbl))  [unwired: 1 in]
              n162 = Bundle By Name("t0"=w254, "dt"=w225, "Y"=w255) -> (→"Bridgewire 2 No-Fire":waveform(dbl))  [unwired: 1 in]
            }
            frame "End BW State" {
              n163 = Enqueue Element(queue=w294, element=LFO_State_Variable."Report") -> ()  [unwired: 2 in, 3 out]
              n164 = property on="stop" class="Bool (strict)"("DisabledEnum"=T11."Disabled and Grayed Out" ("Disabled"), "Value"=FALSE ("Start BW")) -> ()  [unwired: 2 in, 2 out]
              n165 = property on="Reset" class="Bool (strict)"("Visible"=TRUE, "DisabledEnum"=T11."Enabled" ("Disabled"), "Value"=FALSE ("Start BW")) -> ()  [unwired: 2 in, 2 out]
            }
          }
        }
      }
      frame "Report" {
        w308 = "Tested" ("BW1 Dielectric Strength (uA)")
        n166 = local read "BW 1 Insulation Resistance Result"() -> (w312:u16)
        n167 = local read "BW 2 Insulation Resistance Result"() -> (w311:u16)
        n168 = local read "BW 1 Dielectric Strength Result"() -> (w314:u16)
        n169 = local read "BW 2 Dielectric Strength Result"() -> (w313:u16)
        n170 = local read "BW 1 Resistance Result"() -> (w318:u16)
        n171 = local read "BW 2 Resistance Result"() -> (w317:u16)
        n172 = local read "BW 1 No-Fire Result"() -> (w316:u16)
        n173 = local read "BW 2 No-Fire Result"() -> (w315:u16)
        n174 = local read "No-Fire Results BW1"() -> (w334:T6)
        n175 = local read "No-Fire Results BW2"() -> (w335:T6)
        n176 = local read "Raw Data ACW BW2"() -> (w330:T4)
        n177 = local read "Raw Data ACW BW1"() -> (w331:T3)
        n178 = local read "BW 1 Resistance"() -> (w336:string)
        n179 = local read "BW 2 Resistance"() -> (w337:string)
        n180 = local read "BW 2 Results"() -> (w329:T2)
        n181 = local read "BW 1 Results"() -> (w332:T2)
        n182 = Unbundle By Name(w329) -> ("Max Change in Current (A)"=w338:dbl, "Insulation Resistance"=w341:string)
        n183 = Unbundle By Name(w332) -> ("Max Change in Current (A)"=w348:dbl, "Insulation Resistance"=w349:string)
        n184 = Bundle By Name(cluster=T12 {"BW 1 Resistance"="0.7817", "BW 2 Resistance"="1.2990", "No-Fire Results BW1"={"Current"=["7.203409E-06\n", "7.484487E-06\n", "7.484465E-06\n", "8.327806E-06\n", "7.765564E-06\n", "7.062867E-06\n", "8.187235E-06\n", "8.187257E-06\n", "7.906143E-06\n", "7.765622E-06\n", "7.203482E-06\n", "7.484487E-06\n", "7.484487E-06\n", "7.625029E-06\n", "7.765600E-06\n", "7.203387E-06\n", "7.625014E-06\n", "7.765651E-06\n", "8.046671E-06\n", "7.906223E-06\n", "7.343981E-06\n", "7.203409E-06\n", "7.625109E-06\n", "7.765608E-06\n", "7.906143E-06\n", "8.187286E-06\n", "8.046729E-06\n", "7.484501E-06\n", "8.046707E-06\n", "7.906157E-06\n", "7.484501E-06\n", "7.062881E-06\n", "7.906165E-06\n", "7.625087E-06\n", "7.906179E-06\n", "7.765622E-06\n", "7.765593E-06\n", "7.343951E-06\n", "7.906230E-06\n", "7.625087E-06\n", "7.062867E-06\n", "7.484530E-06\n", "7.906172E-06\n", "7.906157E-06\n", "7.625029E-06\n", "7.906143E-06\n", "7.625073E-06\n", "7.343959E-06\n", "8.187249E-06\n", "8.187220E-06\n", "8.187286E-06\n", "7.906172E-06\n", "7.484487E-06\n", "7.765608E-06\n", "7.625073E-06\n", "7.906172E-06\n", "7.906179E-06\n", "7.484523E-06\n", "7.625051E-06\n", "7.765593E-06\n", "7.484559E-06\n", "7.765637E-06\n", "7.484581E-06\n", "8.046714E-06\n", "7.765630E-06\n", "7.765651E-06\n", "8.187286E-06\n", "8.046707E-06\n", "7.906143E-06\n", "8.046729E-06\n", "7.906143E-06\n", "8.046773E-06\n", "7.625065E-06\n", "7.344046E-06\n", "8.327836E-06\n", "7.765644E-06\n", "7.765630E-06\n", "7.484545E-06\n", "7.765615E-06\n", "7.765644E-06\n", "7.203424E-06\n", "7.906143E-06\n", "7.484523E-06\n", "8.046758E-06\n", "7.765666E-06\n", "7.906165E-06\n", "7.625073E-06\n", "8.327777E-06\n", "7.484523E-06\n", "7.625073E-06\n", "7.906150E-06\n", "7.625065E-06\n", "7.625065E-06\n", "7.765630E-06\n", "7.625124E-06\n", "7.765615E-06\n", "7.484494E-06\n", "7.343966E-06\n", "7.906216E-06\n", "7.765608E-06\n", "7.906194E-06\n", "7.484581E-06\n", "7.765622E-06\n", "7.906208E-06\n", "7.343973E-06\n", "7.062918E-06\n", "7.343981E-06\n", "7.765579E-06\n", "7.484530E-06\n", "7.765637E-06\n", "7.625087E-06\n", "8.046707E-06\n", "8.468349E-06\n", "7.906179E-06\n", "7.625065E-06\n", "7.906150E-06\n", "7.906194E-06\n", "7.765644E-06\n", "7.765622E-06\n", "8.187257E-06\n", "7.484501E-06\n", "7.765608E-06\n", "7.343973E-06\n", "7.906143E-06\n", "7.625051E-06\n", "7.906150E-06\n", "7.765593E-06\n", "7.625044E-06\n", "7.765622E-06\n", "7.625102E-06\n", "7.343959E-06\n", "7.484588E-06\n", "7.765622E-06\n", "7.625109E-06\n", "7.906172E-06\n", "7.343973E-06\n", "7.625102E-06\n", "8.468385E-06\n", "7.906201E-06\n", "7.906194E-06\n", "8.046707E-06\n", "7.625109E-06\n", "7.906172E-06\n", "7.906179E-06\n", "8.046773E-06\n", "7.906216E-06\n", "8.327799E-06\n", "7.906223E-06\n", "7.343995E-06\n", "8.046714E-06\n", "8.046685E-06\n"], "Voltage"=[], "Time"=[]}, "No-Fire Results BW2"={"Current"=["7.203409E-06\n", "7.484487E-06\n", "7.484465E-06\n", "8.327806E-06\n", "7.765564E-06\n", "7.062867E-06\n", "8.187235E-06\n", "8.187257E-06\n", "7.906143E-06\n", "7.765622E-06\n", "7.203482E-06\n", "7.484487E-06\n", "7.484487E-06\n", "7.625029E-06\n", "7.765600E-06\n", "7.203387E-06\n", "7.625014E-06\n", "7.765651E-06\n", "8.046671E-06\n", "7.906223E-06\n", "7.343981E-06\n", "7.203409E-06\n", "7.625109E-06\n", "7.765608E-06\n", "7.906143E-06\n", "8.187286E-06\n", "8.046729E-06\n", "7.484501E-06\n", "8.046707E-06\n", "7.906157E-06\n", "7.484501E-06\n", "7.062881E-06\n", "7.906165E-06\n", "7.625087E-06\n", "7.906179E-06\n", "7.765622E-06\n", "7.765593E-06\n", "7.343951E-06\n", "7.906230E-06\n", "7.625087E-06\n", "7.062867E-06\n", "7.484530E-06\n", "7.906172E-06\n", "7.906157E-06\n", "7.625029E-06\n", "7.906143E-06\n", "7.625073E-06\n", "7.343959E-06\n", "8.187249E-06\n", "8.187220E-06\n", "8.187286E-06\n", "7.906172E-06\n", "7.484487E-06\n", "7.765608E-06\n", "7.625073E-06\n", "7.906172E-06\n", "7.906179E-06\n", "7.484523E-06\n", "7.625051E-06\n", "7.765593E-06\n", "7.484559E-06\n", "7.765637E-06\n", "7.484581E-06\n", "8.046714E-06\n", "7.765630E-06\n", "7.765651E-06\n", "8.187286E-06\n", "8.046707E-06\n", "7.906143E-06\n", "8.046729E-06\n", "7.906143E-06\n", "8.046773E-06\n", "7.625065E-06\n", "7.344046E-06\n", "8.327836E-06\n", "7.765644E-06\n", "7.765630E-06\n", "7.484545E-06\n", "7.765615E-06\n", "7.765644E-06\n", "7.203424E-06\n", "7.906143E-06\n", "7.484523E-06\n", "8.046758E-06\n", "7.765666E-06\n", "7.906165E-06\n", "7.625073E-06\n", "8.327777E-06\n", "7.484523E-06\n", "7.625073E-06\n", "7.906150E-06\n", "7.625065E-06\n", "7.625065E-06\n", "7.765630E-06\n", "7.625124E-06\n", "7.765615E-06\n", "7.484494E-06\n", "7.343966E-06\n", "7.906216E-06\n", "7.765608E-06\n", "7.906194E-06\n", "7.484581E-06\n", "7.765622E-06\n", "7.906208E-06\n", "7.343973E-06\n", "7.062918E-06\n", "7.343981E-06\n", "7.765579E-06\n", "7.484530E-06\n", "7.765637E-06\n", "7.625087E-06\n", "8.046707E-06\n", "8.468349E-06\n", "7.906179E-06\n", "7.625065E-06\n", "7.906150E-06\n", "7.906194E-06\n", "7.765644E-06\n", "7.765622E-06\n", "8.187257E-06\n", "7.484501E-06\n", "7.765608E-06\n", "7.343973E-06\n", "7.906143E-06\n", "7.625051E-06\n", "7.906150E-06\n", "7.765593E-06\n", "7.625044E-06\n", "7.765622E-06\n", "7.625102E-06\n", "7.343959E-06\n", "7.484588E-06\n", "7.765622E-06\n", "7.625109E-06\n", "7.906172E-06\n", "7.343973E-06\n", "7.625102E-06\n", "8.468385E-06\n", "7.906201E-06\n", "7.906194E-06\n", "8.046707E-06\n", "7.625109E-06\n", "7.906172E-06\n", "7.906179E-06\n", "8.046773E-06\n", "7.906216E-06\n", "8.327799E-06\n", "7.906223E-06\n", "7.343995E-06\n", "8.046714E-06\n", "8.046685E-06\n"], "Voltage"=[], "Time"=[]}, "ACW Results BW1"={"ACW Time BW1"=[], "ACW Voltage BW1"=[], "ACW Current BW1"=[]}, "IR Results BW1"={"Max Leakage Current (A)"=0.0, "Min Leakage Current (A)"=0.0, "Max Change in Current (A)"=0.0, "Dielectric Strength Pass?"=FALSE, "Insulation Resistance Pass?"=FALSE, "Insulation Resistance"=""}, "ACW Results BW2"={"ACW Time BW2"=[], "ACW Voltage BW2"=[], "ACW Current BW2"=[]}, "IR Results BW 2"={"Max Leakage Current (A)"=0.0, "Min Leakage Current (A)"=0.0, "Max Change in Current (A)"=0.0, "Dielectric Strength Pass?"=FALSE, "Insulation Resistance Pass?"=FALSE, "Insulation Resistance"=""}} ("Raw Data Results"), "IR Results BW 2"=w329, "IR Results BW1"=w332, "ACW Results BW2"=w330, "ACW Results BW1"=w331, "BW 1 Resistance"=w336, "BW 2 Resistance"=w337, "No-Fire Results BW1"=w334, "No-Fire Results BW2"=w335) -> (w333:T12)
        n185 = Build Array(w318, w317, w316, w315, w314, w313, w312, w311) -> (w310:u16[])
        n186 = Multiply(x=w338, y=1000000.0) -> (x*y=w339:dbl)
        n187 = Multiply(x=w348, y=1000000.0) -> (x*y=w347:dbl)
        n188 = Number To Fractional String(number=w339, precision (6)=i16 1) -> (F-format string=w340:string)  [unwired: 2 in]
        n189 = Fract/Exp String To Number(string=w341) -> (number=w342:dbl)  [unwired: 3 in, 1 out]
        n190 = Number To Fractional String(number=w347, precision (6)=i16 1) -> (F-format string=w351:string)  [unwired: 2 in]
        n191 = Fract/Exp String To Number(string=w349) -> (number=w346:dbl)  [unwired: 3 in, 1 out]
        n192 = local read "Model # Out"() -> (w328:string)
        n193 = local read "Serial # Out"() -> (w327:string)
        n194 = Divide(x=w342, y=1000000.0) -> (x/y=w343:dbl)
        n195 = Divide(x=w346, y=1000000.0) -> (x/y=w345:dbl)
        n196 = local read "base path"() -> (w352:path)
        n197 = Number To Fractional String(number=w343, precision (6)=i16 0) -> (F-format string=w344:string)  [unwired: 2 in]
        n198 = Number To Fractional String(number=w345, precision (6)=i16 1) -> (F-format string=w350:string)  [unwired: 2 in]
        n199 = call "Create Data File.vi"("File Type"=enum16{"text (.txt)", "Excel Workbook (.xlsx)"}."text (.txt)", "base path"=w352, "Description"="Raw", "Serial Number"=w327, "Part Number"=w328) -> ("File Path Out"=w326:path)  [unwired: 5 in, 1 out]
        "Raw Data Path" <- w326
        n200 = Bundle By Name(cluster=T10 {"BW1 Resistance (Ohms)"="4870 ", "BW2 Resistance (Ohms)"="4870 ", "BW1 No-Fire"="4870 ", "BW2 No-Fire"="4870 ", "BW1 Dielectric Strength (uA)"="4870 ", "BW2 Dielectric Strength (uA)"="4870 ", "BW1 Insulation Resistance (MOhms)"="4870 ", "BW2 Insulation Resistance (MOhms)"="4870 "} ("Test Results"), "BW1 Resistance (Ohms)"=w336, "BW2 Resistance (Ohms)"=w337, "BW1 No-Fire"=w308, "BW2 No-Fire"=w308, "BW1 Dielectric Strength (uA)"=w351, "BW2 Dielectric Strength (uA)"=w340, "BW1 Insulation Resistance (MOhms)"=w350, "BW2 Insulation Resistance (MOhms)"=w344) -> (w325:T10)
        n201 = local read "configuration file path"() -> (w324:path)
        n202 = control-ref of="Bridgewire 1 No-Fire"() -> (w323:refnum<vi>)
        n203 = control-ref of="Bridgewire 2 No-Fire"() -> (w322:refnum<vi>)
        n204 = local read "Model # Out"() -> (w320:string)
        n205 = local read "Serial # Out"() -> (w319:string)
        n206 = call "Save Raw Data.vi"("Raw Data Results"=w333, "file path (dialog if empty)"=w326) -> ()  [unwired: 9 in, 1 out]
        n207 = call "Results to Table.vi"("Result Indicators"=w310, "Test Results"=w325, "configuration file path"=w324) -> ("Results Table"=w321:string[][])  [unwired: 7 in, 1 out]
        "Results Table" <- w321
        n208 = local write "Results"(w321) -> ()
        n209 = call "Save LFO Report.vi"("Raw Data Path"=w326, "Bridgewire 2 No-Fire"=w322, "Bridgewire 1 No-Fire"=w323, "Results Table"=w321, "Serial Number"=w319, "Part Number"=w320) -> ()  [unwired: 5 in, 1 out]
      }
      frame "Exit" {
        # "Exit the loop"
      }
    }
  }
  n210 = while {
    shift-right: [w356] -> w5
    shift-left: w17 -> [w362]
    tunnel: w10 -> [w363]
    tunnel: w15 -> [w358]
    tunnel: [w357] -> w13
    tunnel: w2 -> [_]
    stop <- w360 stop-if-true
    # "This loop is the producer loop."
    n211 = event shown="[0] \"Start BW\": Value Change" {
      selector: _ -> [_ _ _ _ _ _ _]
      dyn-events: _ -> [_ _ _ _ _ _ _]
      timeout: 200 -> [_ _ _ _ _ _ _]
      tunnel: w363 -> [w368 w373 w377 _ w386 w418 _]
      tunnel: w362 -> [w367 w372 w376 w380 w387 w417 w431]
      tunnel: [w365 w370 w375 w380 w385 w416 w431] -> w356
      tunnel: [_ _ _ _ w383 w410 FALSE ("stop")] -> w361
      tunnel: w358 -> [w364 w369 w374 w382 w388 _ w434]
      tunnel: [w364 w369 w374 w382 w388 _ w433] -> w357
      event "Start BW": Value Change {
        n212 = event-data() -> ()  [unwired: 1 in, 1 out]
        n213 = Enqueue Element(queue=w368, element=LFO_State_Variable."Bridgewire", error in (no error)=w367) -> (error out=w365:errorcluster)  [unwired: 1 in, 2 out]
      }
      event "Reset": Value Change {
        n214 = event-data() -> ()  [unwired: 1 in, 1 out]
        n215 = Enqueue Element(queue=w373, element=LFO_State_Variable."Reset", error in (no error)=w372) -> (error out=w370:errorcluster)  [unwired: 1 in, 2 out]
      }
      event "Start Vitrek": Value Change {
        n216 = event-data() -> ()  [unwired: 1 in, 1 out]
        n217 = Enqueue Element(queue=w377, element=LFO_State_Variable."ACW and IR Test", error in (no error)=w376) -> (error out=w375:errorcluster)  [unwired: 1 in, 2 out]
      }
      event "stop": Value Change {
        n218 = event-data() -> ()  [unwired: 1 in, 1 out]
        n219 = global write "Door Status Global Variable.vi" "stop"("stop") -> ()
        n220 = local write "Test Status"("Test was aborted by the user" ("Test Status")) -> ()
      }
      event Menu Selection (User) {
        n221 = event-data() -> ("ItemTag"=w384:string)  [unwired: 1 in, 2 out]
        n222 = case shown="\"Exit\", Default" w384 {
          tunnel: w387 -> [w396 w408]
          tunnel: w386 -> [w395 _]
          tunnel: [w394 w407] -> w385
          tunnel: [w393 _] -> w383
          frame "Exit", Default {
            # "Exits the software"
            n223 = Two Button Dialog(message="Are you sure you want to Exit?  ", 1:"No" ("F button name (\"Cancel\")"), 2:"Yes" ("T button name (\"OK\")")) -> (T button?=w389:bool)
            n224 = case shown="False" w389 {
              tunnel: w396 -> [w398 w403]
              tunnel: w395 -> [_ w402]
              tunnel: [w398 w401] -> w394
              tunnel: [FALSE ("stop") TRUE ("stop")] -> w393
              frame False {
              }
              frame True {
                n225 = global write "Door Status Global Variable.vi" "stop"(TRUE ("stop")) -> ()
                n226 = Enqueue Element(queue=w402, element=LFO_State_Variable."Exit", error in (no error)=w403) -> (error out=w401:errorcluster)  [unwired: 1 in, 2 out]
              }
            }
          }
          frame "Save Location" {
            (unwired) path "F:/Departments/Mfg Production/Shares/Plant2/LFO/125332 Electrical Test" ("base path")
            n227 = call "Select Save Location.vi"("error in (no error)"=w408, "Current Save Location"="base path") -> ("error out"=w407:errorcluster, "New Save Location"=w405:path)  [unwired: 8 in]
            n228 = local write "base path"(w405) -> ()
            n229 = global write "Door Status Global Variable.vi" "stop"(TRUE ("stop")) -> ()
          }
        }
      }
      event Panel Close? {
        n230 = event-data() -> ()  [unwired: 1 in, 1 out]
        n231 = Two Button Dialog(message="Are you sure you want to Exit?  ", 1:"No" ("F button name (\"Cancel\")"), 2:"Yes" ("T button name (\"OK\")")) -> (T button?=w412:bool)
        n232 = case shown="False" w412 {
          tunnel: w418 -> [_ w426]
          tunnel: w417 -> [w420 w425]
          tunnel: [w420 w424] -> w416
          tunnel: [TRUE ("Discard?") FALSE ("Discard?")] -> w411
          tunnel: [FALSE ("Discard?") TRUE ("Discard?")] -> w410
          frame False {
          }
          frame True {
            # "Exits the software"
            n233 = global write "Door Status Global Variable.vi" "stop"(TRUE ("stop")) -> ()
            n234 = Enqueue Element(queue=w426, element=LFO_State_Variable."Exit", error in (no error)=w425) -> (error out=w424:errorcluster)  [unwired: 1 in, 2 out]
          }
        }
        n235 = event-data("Discard?"=w411) -> ()  [unwired: 1 in, 1 out]
      }
      event Timeout {
        # "Read status of door here every 200ms"
        n236 = event-data() -> ()  [unwired: 1 in, 1 out]
        n237 = call "Poll Door Status.vi"("task/channels in"=w434) -> ("Cable"=w429:bool, "Door Status"=w432:bool, "task out"=w433:refnum<k21>)  [unwired: 7 in, 1 out]
        n238 = Not(x=w432) -> (.not. x?=w430:bool)
        "Door Status" <- w430
        n239 = global write "Door Status Global Variable.vi" "Cable In Use"(w429) -> ()
        n240 = global write "Door Status Global Variable.vi" "Door Status"(w430) -> ()
      }
    }
    n241 = Or(x=w356, y=w361) -> (x .or. y?=w360:bool)
  }
  n242 = call <vilib>:"Clear Errors.vi"("error in (no error)"=w5) -> ("error out"=w4:errorcluster)  [unwired: 5 in, 1 out]
  n243 = call <vilib>:"DAQmx Stop Task.vi"("task/channels in"=w13, "error in"=w4) -> ("error out"=w12:errorcluster)  [unwired: 12 in, 1 out]
  n244 = Release Queue(queue=w10, error in (no error)=w12) -> (error out=w3:errorcluster)  [unwired: 1 in, 2 out]
  n245 = disable-structure shown="RUN_TIME_ENGINE==True" {
    disable-tunnel: w3 -> [_ _]
    frame condition #0 {
      n246 = Quit LabVIEW() -> ()  [unwired: 1 in]
    }
    frame condition #1 (active) {
    }
  }
